vi "WaterTank.vi"() -> ()   [LabVIEW 2018]
panel:
  out "Water Tank":dbl(slide) scale=0.0..100.0
  out "Tube 14":bool
  in  "Valve 4":bool
  out "Tube 13":bool
  out "Tube 6":bool
  out "Tube 5":bool
  out "Tube 4":bool
  out "Tube 3":bool
  out "Tube 2":bool
  in  "valve 1":bool
  out "Tube 1":bool
  out "Pump 1":bool
  in  "Motor":bool
  in  "stop":bool
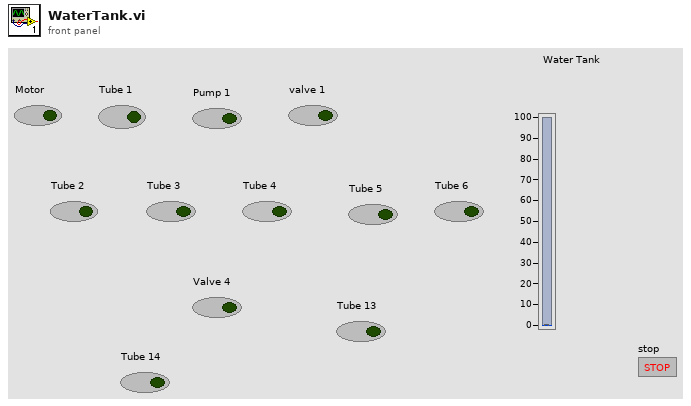
[diagram p1: front panel]
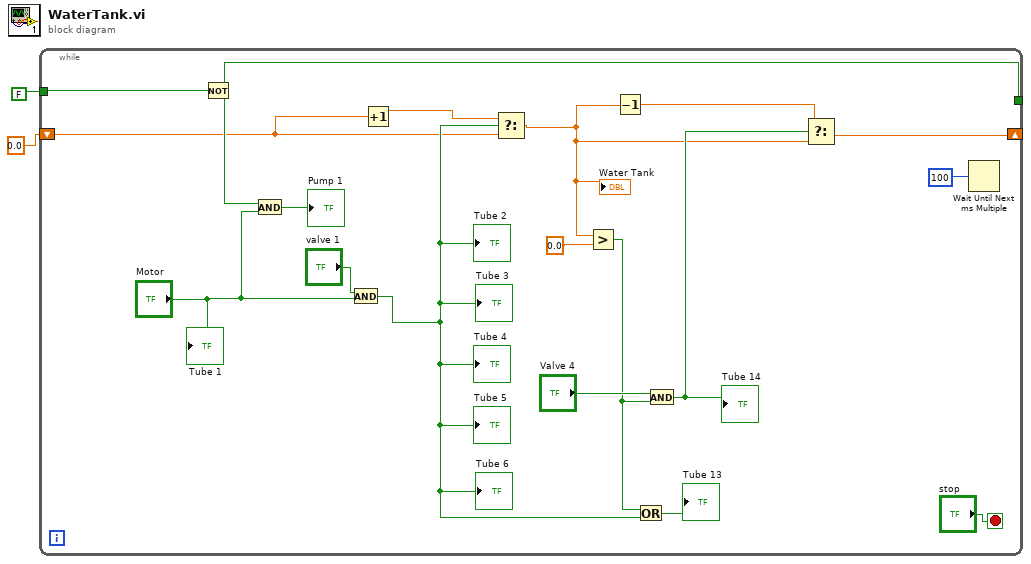
[diagram p0: block diagram]
diagram:
  n1 = while {
    tunnel: [w18] -> _
    tunnel: FALSE -> [w9]
    shift-right: [w3] -> _
    shift-left: 0.0 -> [w4]
    stop <- "stop" stop-if-true
    n2 = Not(x=w9) -> (.not. x?=w18:bool)
    n3 = And(x=w18, y="Motor") -> (x .and. y?=→"Pump 1":bool)
    n4 = And(x="valve 1", y="Motor") -> (x .and. y?=w7:bool)
    "Tube 2" <- w7
    "Tube 3" <- w7
    "Tube 4" <- w7
    "Tube 5" <- w7
    "Tube 6" <- w7
    n5 = Increment(x=w4) -> (x+1=w20:dbl)
    n6 = Select(t=w20, s=w7, f=w4) -> (s? t:f=w5:dbl)
    "Water Tank" <- w5
    n7 = Greater?(x=w5, y=0.0) -> (0:w11:bool)
    n8 = Decrement(x=w5) -> (x-1=w13:dbl)
    n9 = Or(x=w11, y=w7) -> (x .or. y?=→"Tube 13":bool)
    n10 = And(x="Valve 4", y=w11) -> (x .and. y?=w10:bool)
    "Tube 14" <- w10
    n11 = Select(t=w13, s=w10, f=w5) -> (s? t:f=w3:dbl)
    n12 = Wait Until Next ms Multiple(millisecond multiple=100) -> ()  [unwired: 1 out]
    "Tube 1" <- "Motor"
  }
